vi "EF_GetFeaturesVectorAutoregression.vi"(8 "error in (no error)":errorcluster, 10 "AR order":i32=4, 11 "Array Of Waveforms in":waveform(dbl)[](array[waveform])) -> (0 "error out":errorcluster, 3 "Features Array out":dbl[][](array[numeric]))   [LabVIEW 2016, in "Feature Extraction.lvlib"]
uses:
  <vilib>/addons/Time Series Analysis/Modeling and Prediction.llb/TSA Vector AR Modeling (Waveform).vi
  Feature Extraction.lvlib
  <vilib>/addons/_Advanced Signal Processing/NI_AdvSigProcTSA.lvlib
panel:
  # "This VI is a part of BCI Design library, http://www.ru-bci.org \nCopyright © 2020, Sotnikov Peter, All rights reserved. License: GNU GPLv3"
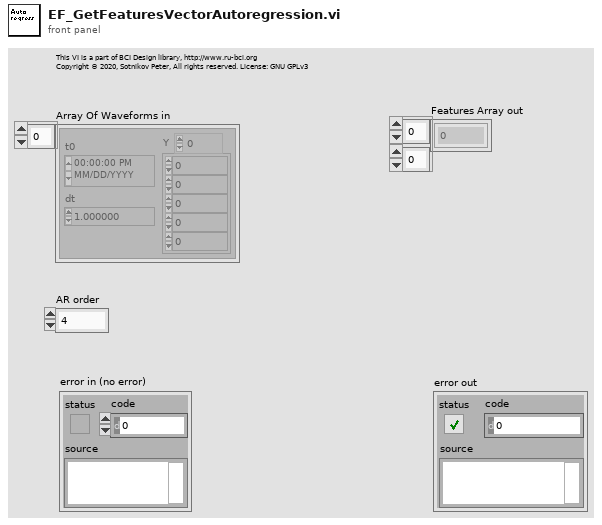
[diagram p1: front panel]
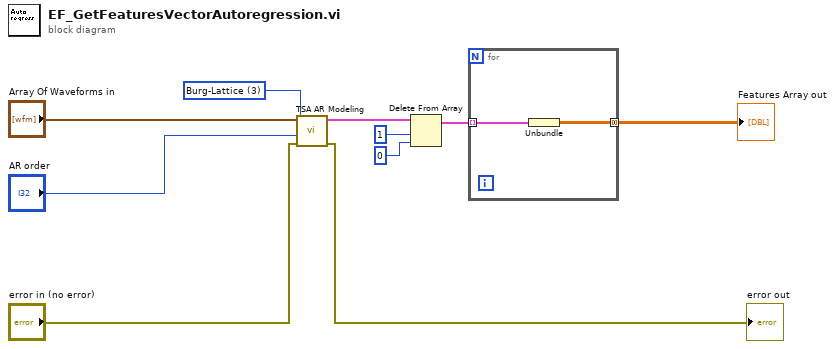
[diagram p0: block diagram]
diagram:
  w7 = u16 3 items=["Forward-Backward", "Least-Squares", "Yule-Walker", "Burg-Lattice", "Geometric-Lattice"] ("AR method")
  n1 = call-poly <vilib>:"TSA AR Modeling.vi"("error in (no error)"="error in (no error)", "AR order"="AR order", "AR method"=w7, "Xt"="Array Of Waveforms in") -> ("error out"=→"error out":errorcluster, "AR coefficients"=w6:cluster{dbl[][]}[])  [unwired: 5 in, 1 out]
  n2 = Delete From Array(array=w6, length=1, index=0) -> (array with subset deleted=w3:cluster{dbl[][]}[])  [unwired: 1 out]
  n3 = for {
    tunnel: w3 -> [w12] mode=indexing
    tunnel: [w11] -> w2 mode=concatenating
    n4 = Unbundle(w12) -> (w11:dbl[][])
  }
  "Features Array out" <- w2
